vi "search for item.vi"(8 "error in (no error)":errorcluster, 10 "Name in bitfile":string, 11 "FPGA Resources in":T1[](array[typedef])) -> (0 "error out":errorcluster, 1 "index of element":i32, 2 "FPGA Resource":T1)   [LabVIEW 2016, in "FPGA Resource Manager System Definition.lvlib"]
uses:
  FPGA Resource Manager System Definition.lvlib
  FPGA-Addon/Source/System Explorer/SubVIs/fpga resource.ctl
  FPGA-Addon/Source/System Explorer/SubVIs/Channel Type.ctl
  FPGA-Addon/Source/System Explorer/FPGA Addon System Explorer.lvlib
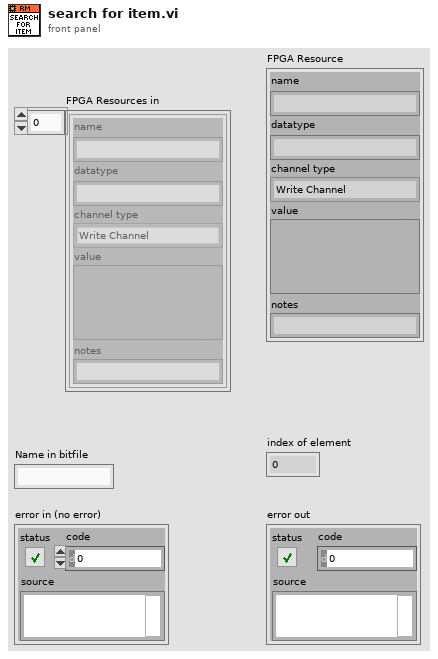
[diagram p1: front panel]
types:
  T1 = typedef "FPGA Addon System Explorer.lvlib/fpga resource.ctl" = cluster{"name":string, "datatype":string, "channel type":T2, "value":variant, "notes":string}
  T2 = typedef "FPGA Addon System Explorer.lvlib/Channel Type.ctl" = enum16{"Write Channel", "Read Channel", "Write Waveform", "Read Waveform"}
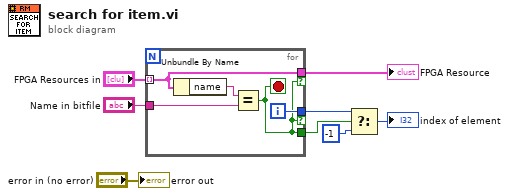
[diagram p0: block diagram]
diagram:
  n1 = for {
    tunnel: "FPGA Resources in" -> [w11] mode=indexing
    tunnel: "Name in bitfile" -> [w12]
    tunnel: [w11] -> w7 if=w9
    tunnel: [w10] -> w5 if=w9
    tunnel: [w9] -> w6
    i -> [w10]
    stop <- w9 stop-if-true
    n2 = Unbundle By Name(w11) -> ("name"=w13:string)
    n3 = Equal?(x=w13, y=w12) -> (x = y?=w9:bool)
  }
  "FPGA Resource" <- w7
  n4 = Select(t=w5, s=w6, f=-1) -> (s? t:f=→"index of element":i32)
  "error out" <- "error in (no error)"
